vi "ConfigMCSS.vi"(6 "Channel Names":string[](array[string]), 8 "error in":errorcluster, 9 "maximum value":dbl=0.01 format="%^.2e", 10 "minimum value":dbl=-0.01 format="%^.2e", 11 "DAQmx Physical Channels":tag[](array[tag])) -> (0 "error out":errorcluster, 3 "DAQmx Task Name":refnum<k21>)   [LabVIEW 2025]
uses:
  <vilib>/DAQmx/create/channels.llb/DAQmx Create Channel (AI-Voltage-Basic).vi
  <vilib>/DAQmx/configure/timing.llb/DAQmx Timing (Sample Clock).vi
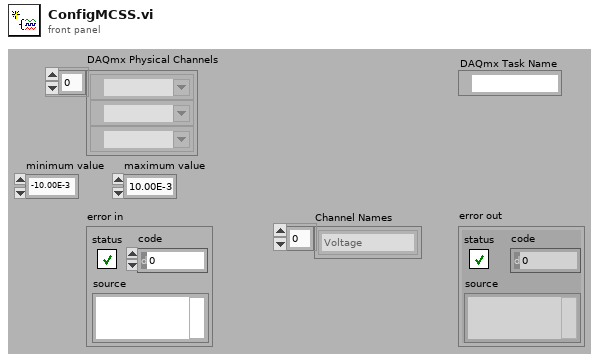
[diagram p1: front panel]
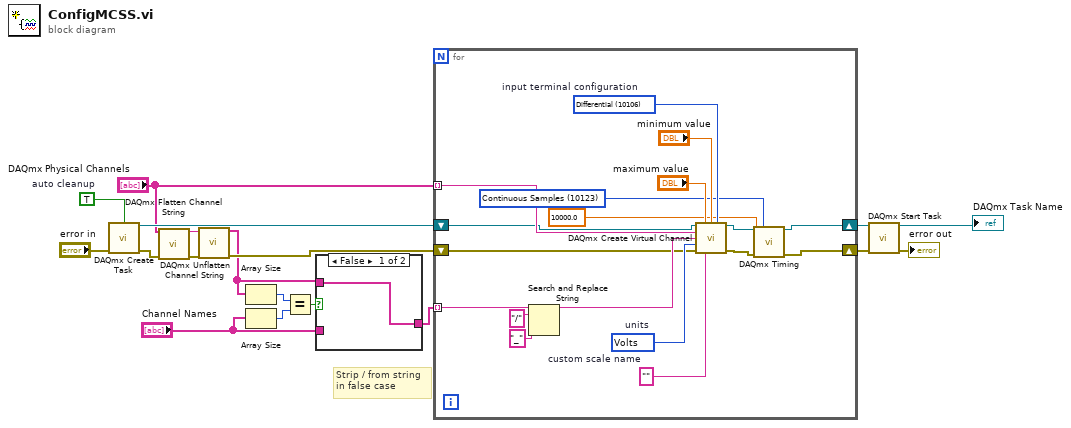
[diagram p0: block diagram]
diagram:
  w17 = TRUE  # auto cleanup
  # "Strip / from string\nin false case"
  n1 = call <vilib>:"DAQmx Create Task.vi"("auto cleanup"=w17, "error in"="error in") -> ("task out"=w16:refnum<k21>, "error out"=w9:errorcluster)  [unwired: 12 in]
  n2 = call <vilib>:"DAQmx Flatten Channel String.vi"("names in"="DAQmx Physical Channels", "error in"=w9) -> ("names out"=w11:string, "error out"=w10:errorcluster)  [unwired: 12 in]
  n3 = call <vilib>:"DAQmx Unflatten Channel String.vi"("names in"=w11, "error in"=w10) -> ("names out"=w1:string[], "error out"=w8:errorcluster)  [unwired: 12 in]
  n4 = Array Size(array=w1) -> (size(s)=w15:i32)
  n5 = Array Size(array="Channel Names") -> (size(s)=w14:i32)
  n6 = Equal?(x=w15, y=w14) -> (x = y?=w13:bool)
  n7 = case shown="False" w13 {
    tunnel: [w19 w20] -> w2
    tunnel: "Channel Names" -> [_ w20]
    tunnel: w1 -> [w19 _]
    frame False {
    }
    frame True {
    }
  }
  n8 = for {
    tunnel: w2 -> [w29] mode=indexing
    shift-right: [w22] -> w5
    shift-left: w8 -> [w25]
    shift-right: [w21] -> w7
    shift-left: w16 -> [w26]
    tunnel: "DAQmx Physical Channels" -> [w33] mode=indexing
    w27 = 10123 items=["Finite Samples"=10178, "Continuous Samples"=10123, "Hardware Timed Single Point"=12522] ("sample mode")
    w34 = 10106 items=["default"=-1, "RSE"=10083, "NRSE"=10078, "Differential"=10106, "Pseudodifferential"=12529]  # input terminal configuration
    w35 = 10348 items=["Volts"=10348, "From Custom Scale"=10065]  # units
    w36 = ""  # custom scale name
    n9 = Search and Replace String(input string=w29, search string="/", replace string="_" ("replace string (\"\")")) -> (result string=w30:string)  [unwired: 5 in, 3 out]
    n10 = call-poly <vilib>:"DAQmx Create Virtual Channel.vi"("task in"=w26, "maximum value"="maximum value", "minimum value"="minimum value", "input terminal configuration"=w34, "physical channels"=w33, "name to assign"=w30, "units"=w35, "error in"=w25, "custom scale name"=w36) -> ("task out"=w24:refnum<k21>, "error out"=w23:errorcluster)  [unwired: 5 in]
    n11 = call-poly <vilib>:"DAQmx Timing.vi"("task/channels in"=w24, "sample mode"=w27, "rate"=10000.0, "error in"=w23) -> ("task out"=w21:refnum<k21>, "error out"=w22:errorcluster)  [unwired: 10 in]
  }
  n12 = call <vilib>:"DAQmx Start Task.vi"("task/channels in"=w7, "error in"=w5) -> ("task out"=→"DAQmx Task Name":refnum<k21>, "error out"=→"error out":errorcluster)  [unwired: 12 in]
